vi "Get Array Elements (by Offset).vi"(6 "Pass non-arrays":bool, 8 "error in (no error)":errorcluster, 10 "Offset":i32, 11 "JSON":string) -> (0 "error out":errorcluster, 1 "Element Offsets":i32[](array[numeric]), 2 "Offset past":i32 caption="Offset past Array", 4 "Element End Offsets":i32[](array[numeric]))   [LabVIEW 2024, in "JSONtext.lvlib"]
doc: "If a JSON Array, returns all elements of the Array.\n\nIf the input JSON is not an Array, this function will return an error, unless \"Pass non-arrays\" is true, in which case the output will be a one-element array containing the input JSON."
uses:
  JSONtext.lvlib
  Parsing State.ctl
  Advance past Line Ending.vi
  Advance past String.vi
  Advance past Number.vi
  Advance past Array.vi
  Advance past Object.vi
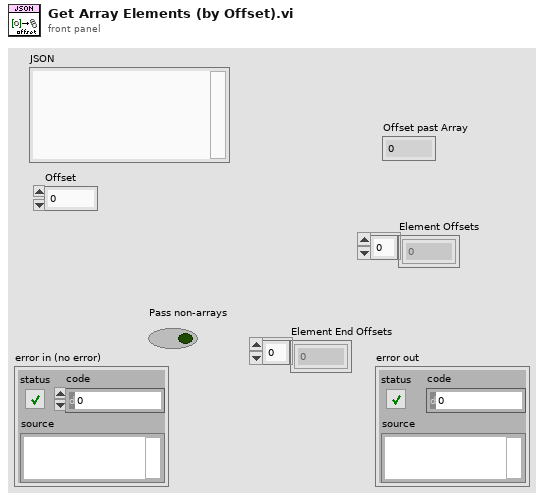
[diagram p1: front panel]
types:
  T1 = typedef "JSONtext.lvlib/Parsing State.ctl" = enum16{"Parser Error", "Object", "Array", "String", "Number/Other", "Leading Whitespace", "Object end", "Array end", "Value end"}
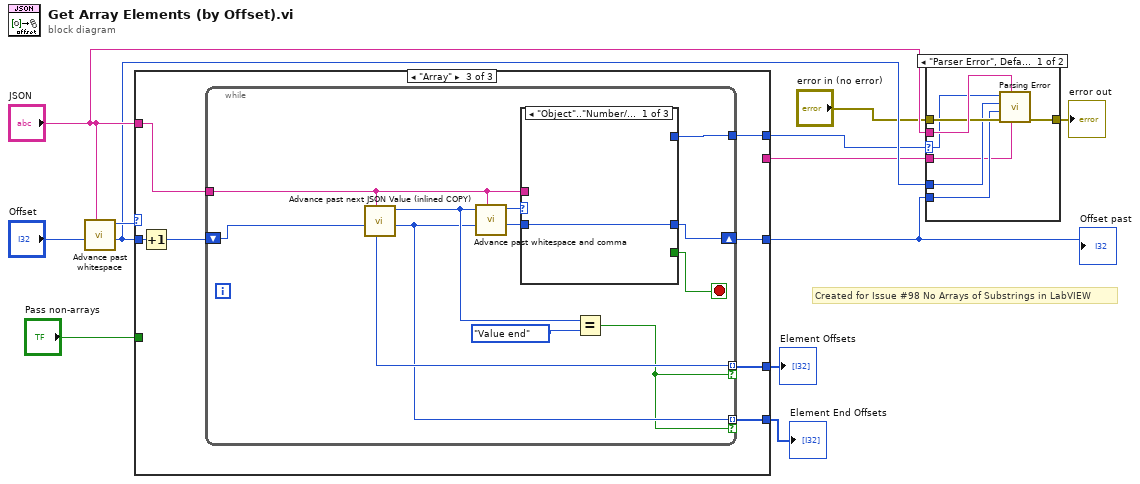
[diagram p0: block diagram]
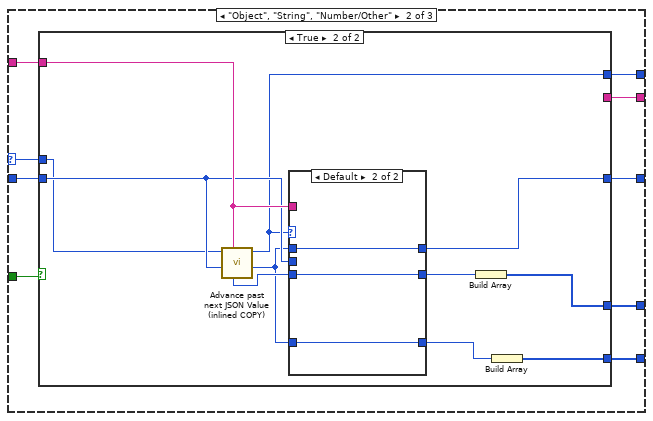
[diagram p4: hidden frame]
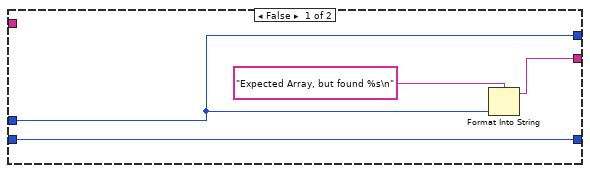
[diagram p5: hidden frame]
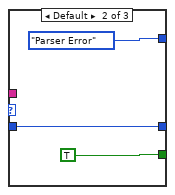
[diagram p7: hidden frame]
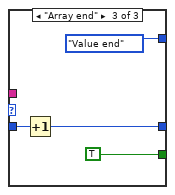
[diagram p8: hidden frame]
diagram:
  # "Created for Issue #98 No Arrays of Substrings in LabVIEW"
  n1 = call "Advance past whitespace.vi"("JSON"="JSON", "Offset"="Offset") -> ("Offset of first non-whitespace"=w9:i32, "Parser State"=w11:T1)  [unwired: 7 in, 1 out]
  n2 = case shown="\"Array\"" w11 {
    selector: w11 -> [w14 w17 _]
    tunnel: [w14 w19 w49] -> w5
    tunnel: [w13 w20 w48] -> w8
    tunnel: [_ w21 w46] -> w2
    tunnel: "JSON" -> [_ w23 w45]
    tunnel: w9 -> [w13 w22 w44]
    tunnel: "Pass non-arrays" -> [_ w18 _]
    tunnel: [_ w16 _] -> w3
    tunnel: [_ w15 w43] -> w1
    frame "Parser Error", Default {
    }
    frame "Object", "String", "Number/Other" {
      n3 = case shown="True" w18 {
        tunnel: w23 -> [_ w38]
        tunnel: w22 -> [w27 w37]
        tunnel: [_ w34] -> w21
        tunnel: [w27 w33] -> w20
        tunnel: [w25 w32] -> w19
        tunnel: w17 -> [w25 w31]
        tunnel: [w24 _] -> w16
        tunnel: [_ w28] -> w15
        frame False {
          n4 = Format Into String(format string="Expected Array, but found %s\n", w25) -> (resulting string=w24:string)  [unwired: 2 in, 1 out]
        }
        frame True {
          n5 = call "Advance past next JSON Value (inlined COPY).vi"("JSON"=w38, "Offset"=w37, "State"=w31) -> ("Offset"=w29:i32, "State"=w32:T1, "Value start"=w36:i32)  [unwired: 4 in, 2 out]
          n6 = case shown="Default" w32 {
            tunnel: w36 -> [_ w41]
            tunnel: w37 -> [_ _]
            tunnel: w29 -> [w39 w42]
            tunnel: [_ w41] -> w35
            tunnel: w38 -> [_ _]
            tunnel: [w39 w42] -> w33
            tunnel: [_ w40] -> w30
            tunnel: w29 -> [_ w40]
            frame "Parser Error" {
            }
            frame Default {
            }
          }
          n7 = Build Array(w35) -> (w34:i32[])
          n8 = Build Array(w30) -> (w28:i32[])
        }
      }
    }
    frame "Array" {
      n9 = Increment(x=w44) -> (x+1=w47:i32)
      n10 = while {
        tunnel: w45 -> [w55]
        shift-right: [w58] -> w48
        shift-left: w47 -> [w59]
        tunnel: [w56] -> w49
        tunnel: [w52] -> w46 mode=indexing if=w50
        tunnel: [w51] -> w43 mode=indexing if=w50
        stop <- w57 stop-if-true
        n11 = call "Advance past next JSON Value (inlined COPY).vi"("JSON"=w55, "Offset"=w59) -> ("Offset"=w51:i32, "State"=w53:T1, "Value start"=w52:i32)  [unwired: 5 in, 2 out]
        n12 = call "Advance past whitespace and comma.vi"("JSON"=w55, "Offset"=w51, "State in"=w53) -> ("Offset past match"=w61:i32, "State"=w60:T1)  [unwired: 6 in, 1 out]
        n13 = case shown="\"Object\"..\"Number/Other\"" w60 {
          tunnel: [_ TRUE TRUE] -> w57
          tunnel: [_ Parsing_State."Parser Error" Parsing_State."Value end"] -> w56
          tunnel: w61 -> [w62 w63 w67]
          tunnel: [w62 w63 w66] -> w58
          tunnel: w55 -> [_ _ _]
          frame "Object".."Number/Other" {
          }
          frame Default {
          }
          frame "Array end" {
            n14 = Increment(x=w67) -> (x+1=w66:i32)
          }
        }
        n15 = Equal?(x=w53, y=Parsing_State."Value end") -> (x = y?=w50:bool)
      }
    }
  }
  "Offset past" <- w8
  "Element Offsets" <- w2
  "Element End Offsets" <- w1
  n16 = case shown="\"Parser Error\", Default" w5 {
    selector: w5 -> [w71 _]
    tunnel: "JSON" -> [w76 _]
    tunnel: "error in (no error)" -> [w75 w77]
    tunnel: [w74 w77] -> w7
    tunnel: w9 -> [w73 _]
    tunnel: w8 -> [w72 _]
    tunnel: w3 -> [w70 _]
    frame "Parser Error", Default {
      n17 = call "Parsing Error.vi"("initial string"=w70, "JSON"=w76, "error in (no error)"=w75, "Offset past match"=w72, "Value start"=w73, "State"=w71) -> ("error out"=w74:errorcluster)  [unwired: 5 in]
    }
    frame "Value end" {
    }
  }
  "error out" <- w7
